vi "Gen Stage 2 Update gRPC.vi"(7 "Staus":refnum<vi>, 8 "error in":errorcluster, 10 "New Subname":string, 11 "Template Project Path":path) -> (0 "error out":errorcluster, 1 "Proto Names":T1)   [LabVIEW 2021, in "Plugin Generator.lvlib"]
uses:
  Plugin Generator.lvlib
  Typedef/Proto Names.ctl
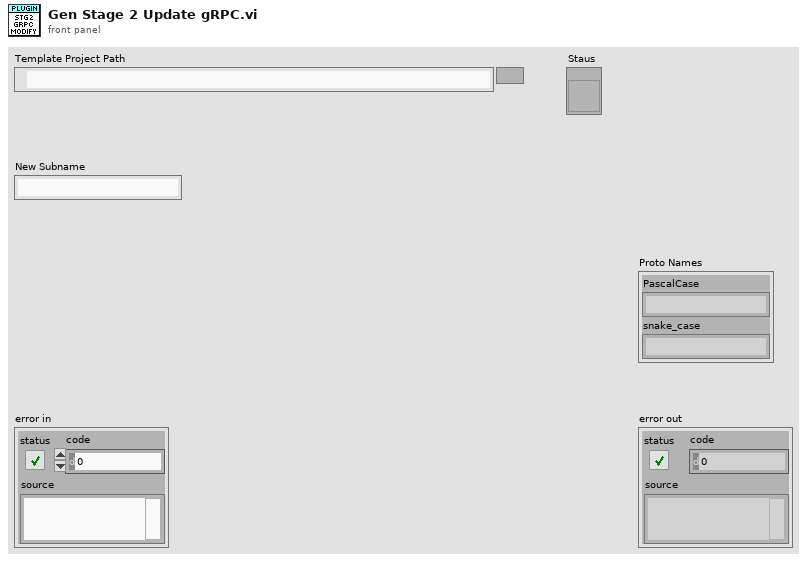
[diagram p1: front panel]
types:
  T1 = typedef "Plugin Generator.lvlib/Proto Names.ctl" = cluster{"PascalCase":string, "snake_case":string}
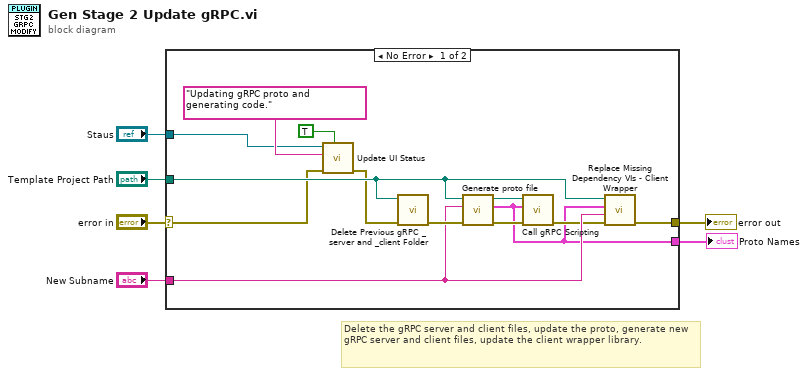
[diagram p0: block diagram]
diagram:
  # "Delete the gRPC server and client files, update the proto, generate new gRPC server and client files, update the client wrapper library."
  n1 = case shown="No Error" "error in" {
    selector: "error in" -> [w9 w20]
    tunnel: [w19 w20] -> w6
    tunnel: "New Subname" -> [w14 _]
    tunnel: "Template Project Path" -> [w15 _]
    tunnel: [w12 _] -> w2
    tunnel: "Staus" -> [w10 _]
    frame No Error {
      n2 = call "Update UI Status.vi"("Previous Complete"=TRUE, "error in"=w9, "Status to Display"="Updating gRPC proto and generating code." ("To display"), "String in"=w10) -> ("error out"=w8:errorcluster)  [unwired: 7 in]
      n3 = call "Delete Previous gRPC _server and _client Folder.vi"("error in"=w8, "Template Project Path"=w15) -> ("error out"=w16:errorcluster)  [unwired: 9 in]
      n4 = call "Generate proto file.vi"("error in"=w16, "New Subname"=w14, "Template Project Path"=w15) -> ("error out"=w18:errorcluster, "Proto Names"=w12:T1, "proto File Path"=w17:path)  [unwired: 6 in]
      n5 = call "Call gRPC Scripting.vi"("error in"=w18, "Proto Names"=w12, "proto File Path"=w17) -> ("error out"=w13:errorcluster)  [unwired: 8 in]
      n6 = call "Replace Missing Dependency VIs - Client Wrapper.vi"("error in"=w13, "New Subname"=w14, "Proto Names"=w12, "Template Project Path"=w15) -> ("error out"=w19:errorcluster)  [unwired: 7 in]
    }
    frame Error {
    }
  }
  "error out" <- w6
  "Proto Names" <- w2
